vi "DSF.Engine.BuilderManager.Initialize.vi"(7 "Framework Cache":refnum<class "DSF.Engine.Memory.Cache.Framework.lvclass">, 8 "error in (no error)":errorcluster, 11 "Builder Manager in":refnum<class "DSF.Engine.BuilderManager.lvclass">) -> (0 "error out":errorcluster, 3 "Builder Manager out":refnum<class "DSF.Engine.BuilderManager.lvclass">)   [LabVIEW 2016, in "DSF.Engine.lvlib" / "DSF.Engine.BuilderManager.lvclass"]
uses:
  DSF.Engine.BuilderManager.lvclass
  Cache/DSF.Engine.Memory.Cache.Framework.lvclass
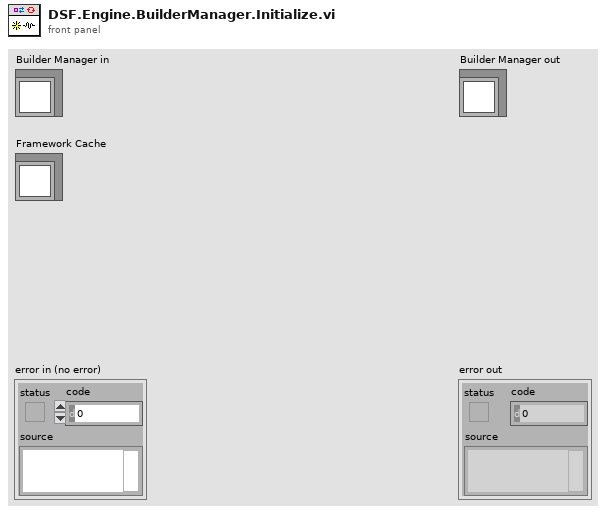
[diagram p1: front panel]
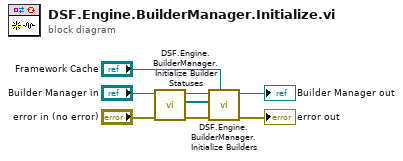
[diagram p0: block diagram]
diagram:
  n1 = call "DSF.Engine.BuilderManager.Initialize Builder Statuses.vi"("error in (no error)"="error in (no error)", "Builder Manager in"="Builder Manager in") -> ("error out"=w4:errorcluster, "Builder Statuses"=w3:refnum<class "Status.Builder.lvclass">[], "Builder Manager out"=w6:refnum<class "DSF.Engine.BuilderManager.lvclass">)  [unwired: 7 in]
  n2 = call "DSF.Engine.BuilderManager.Initialize Builders.vi"("Framework Cache"="Framework Cache", "error in (no error)"=w4, "Builder Statuses"=w3, "Builder Manager in"=w6) -> ("error out"=→"error out":errorcluster, "Builder Manager out"=→"Builder Manager out":refnum<class "DSF.Engine.BuilderManager.lvclass">)  [unwired: 6 in]
